vi "reference point (SubVI).vi"(0 "Nb Circles (Circle Detection 1)":i32, 1 "Straight Edge (Find Straight Edge 1)":T1, 2 "Straight Edge (Find Straight Edge 2)":T1, 3 "Particle Measurements (Real-World) (Particle Analysis 1)":dbl[][](array[numeric]) format="%.2f") -> (5 "Puck X, Y co-ordinates":dbl[][](array[numeric]), 6 "Player X, Y co-ordinates":dbl[][](array[numeric]))   [LabVIEW 2013]
uses:
  <vilib>/vision/NI_Vision_Development_Module.lvlib
panel:
  out "Reference Point in real\n (intersection)":cluster{"X":sgl, "Y":sgl} {"Y" format="%.2f"; "X" format="%.2f"}
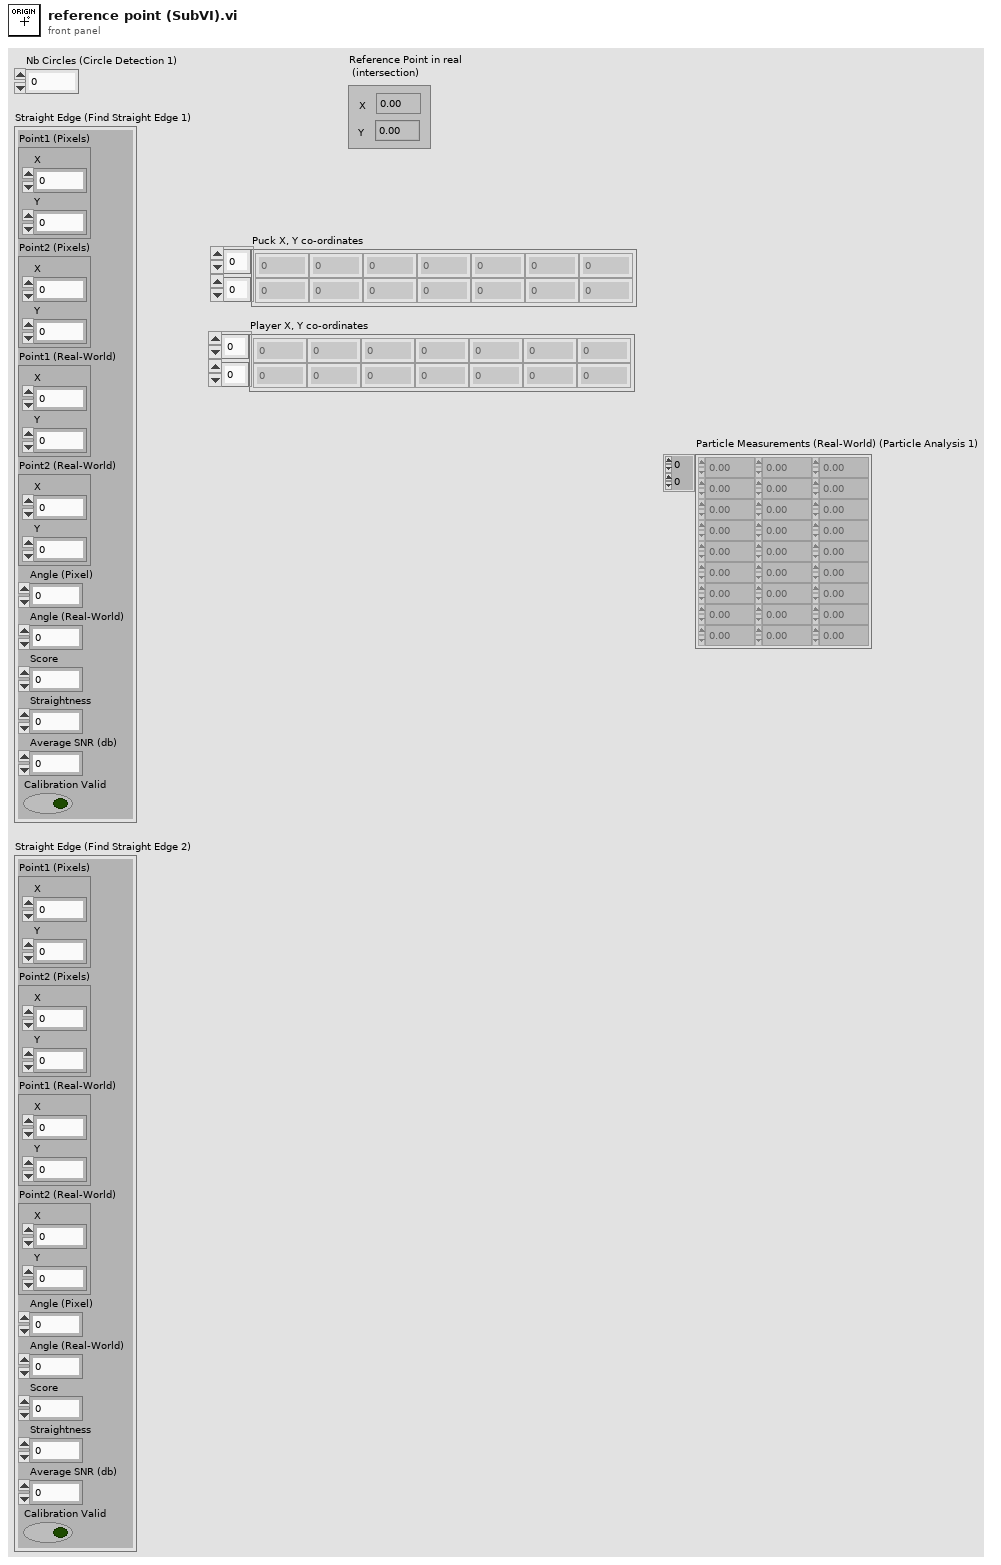
[diagram p1: front panel]
types:
  T1 = cluster{"Point1 (Pixels)":cluster{"X":sgl, "Y":sgl}, "Point2 (Pixels)":cluster{"X":sgl, "Y":sgl}, "Point1 (Real-World)":cluster{"X":sgl, "Y":sgl}, "Point2 (Real-World)":cluster{"X":sgl, "Y":sgl}, "Angle (Pixel)":dbl, "Angle (Real-World)":dbl, "Score":dbl, "Straightness":dbl, "Average SNR (db)":dbl, "Calibration Valid":bool}
  T2 = cluster{"Point1 (Real-World)":cluster{"X":sgl, "Y":sgl}, "Point2 (Real-World)":cluster{"X":sgl, "Y":sgl}}
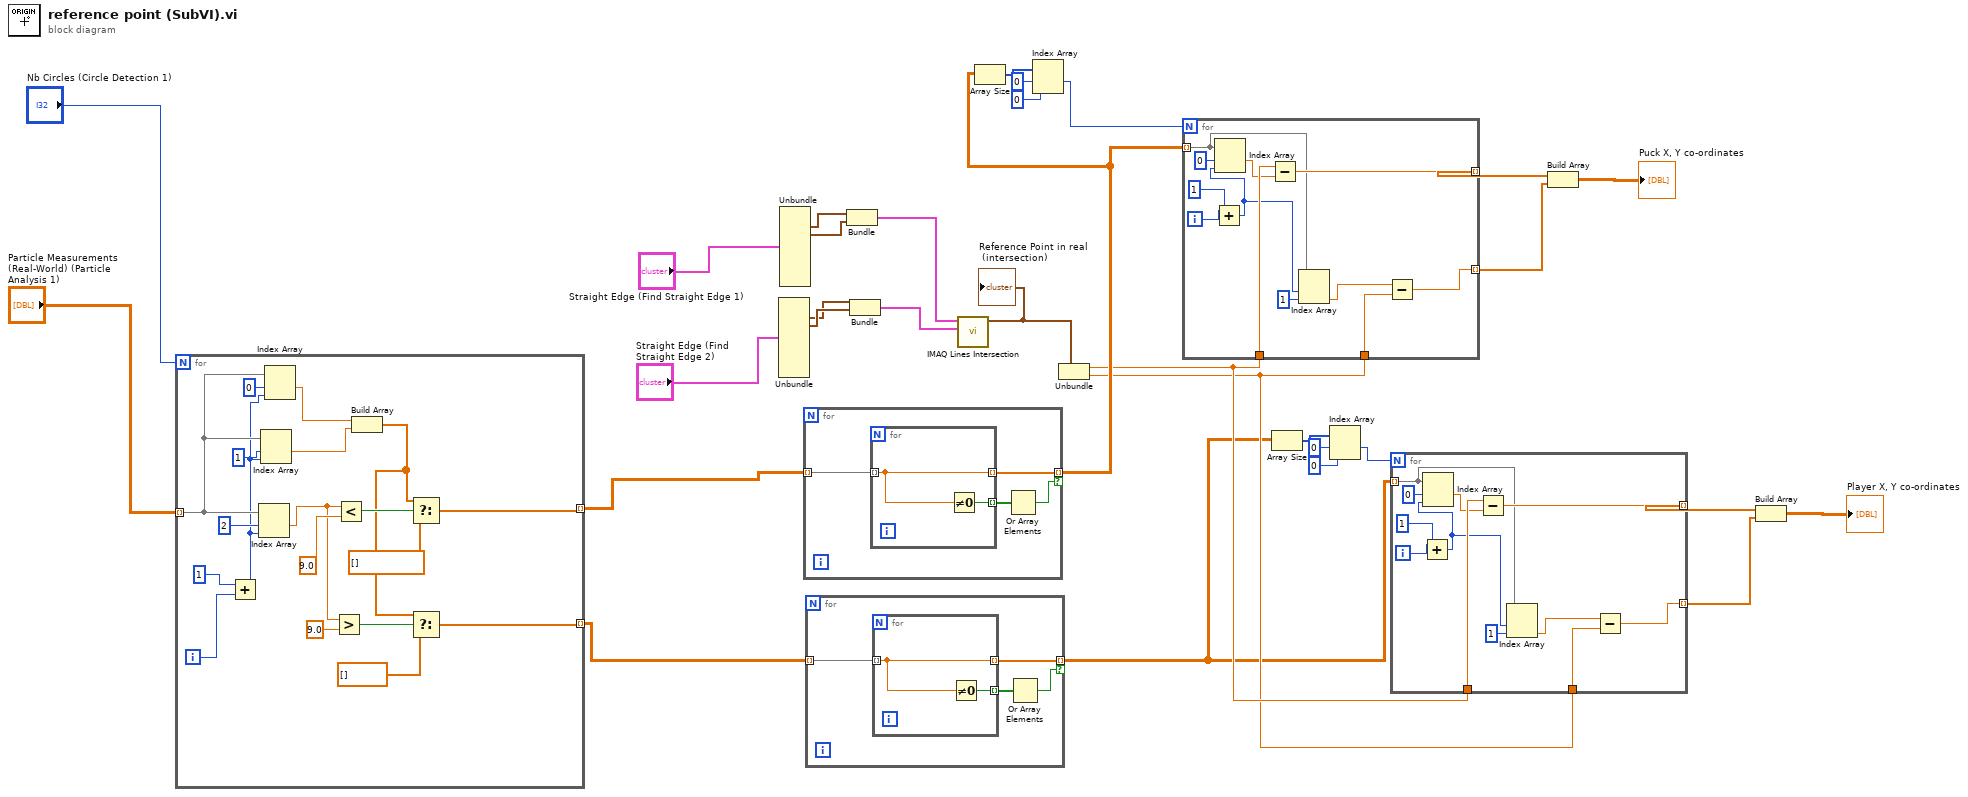
[diagram p0: block diagram]
diagram:
  n1 = for {
    N: "Nb Circles (Circle Detection 1)" -> [_]
    tunnel: "Particle Measurements (Real-World) (Particle Analysis 1)" -> [w43] mode=indexing
    tunnel: [w45] -> w18 mode=indexing
    tunnel: [w32] -> w17 mode=indexing
    i -> [w49]
    n2 = Add(x=1, y=w49) -> (x+y=w41:i32)
    n3 = Index Array(array=w43, index #1=2 ("index"), index #2=w41) -> (element #1=w36:dbl)  [unwired: 1 out]
    n4 = Index Array(array=w43, index #1=1 ("index"), index #2=w41) -> (element #1=w39:dbl)  [unwired: 1 out]
    n5 = Index Array(array=w43, index #1=0 ("index"), index #2=w41) -> (element #1=w40:dbl)  [unwired: 1 out]
    n6 = Greater?(x=w36, y=9.0) -> (0:w35:bool)
    n7 = Less?(x=w36, y=9.0) -> (x < y?=w46:bool)
    n8 = Build Array(w40, w39) -> (w34:dbl[])
    n9 = Select(t=w34, s=w46, f=dbl[] []) -> (s? t:f=w45:dbl[])
    n10 = Select(t=w34, s=w35, f=dbl[] []) -> (s? t:f=w32:dbl[])
  }
  n11 = Unbundle("Straight Edge (Find Straight Edge 2)") -> ("Point1 (Real-World)"=w23:cluster{"X":sgl, "Y":sgl}, "Point2 (Real-World)"=w24:cluster{"X":sgl, "Y":sgl})  [unwired: 8 out]
  n12 = Unbundle("Straight Edge (Find Straight Edge 1)") -> ("Point1 (Real-World)"=w26:cluster{"X":sgl, "Y":sgl}, "Point2 (Real-World)"=w25:cluster{"X":sgl, "Y":sgl})  [unwired: 8 out]
  n13 = for {
    tunnel: w18 -> [w54] mode=indexing
    tunnel: [w52] -> w15 mode=indexing if=w51
    n14 = for {
      tunnel: w54 -> [w55] mode=indexing
      tunnel: [w56] -> w53 mode=indexing
      tunnel: [w55] -> w52 mode=indexing
      n15 = Not Equal To 0?(x=w55) -> (x != 0?=w56:bool)
    }
    n16 = Or Array Elements(Boolean array=w53) -> (logical OR=w51:bool)
  }
  n17 = for {
    tunnel: w17 -> [w60] mode=indexing
    tunnel: [w58] -> w1 mode=indexing if=w57
    n18 = for {
      tunnel: w60 -> [w61] mode=indexing
      tunnel: [w62] -> w59 mode=indexing
      tunnel: [w61] -> w58 mode=indexing
      n19 = Not Equal To 0?(x=w61) -> (x != 0?=w62:bool)
    }
    n20 = Or Array Elements(Boolean array=w59) -> (logical OR=w57:bool)
  }
  n21 = Bundle("Point1 (Real-World)"=w26, "Point2 (Real-World)"=w25) -> (w30:T2)  [unwired: 1 in]
  n22 = Bundle("Point1 (Real-World)"=w23, "Point2 (Real-World)"=w24) -> (w28:T2)  [unwired: 1 in]
  n23 = call "IMAQ Lines Intersection"("Line 2"=w28, "Line 1"=w30) -> ("Intersection Point"=w31:cluster{"X":sgl, "Y":sgl})  [unwired: 7 in, 2 out]
  "Reference Point in real\n (intersection)" <- w31
  n24 = Array Size(array=w15) -> (size(s)=w14:i32[])
  n25 = Index Array(array=w14, index #1=0 ("index"), index #2=0 ("index")) -> (element #1=w11:i32)  [unwired: 1 out]
  n26 = Unbundle(w31) -> ("X"=w7:sgl, "Y"=w6:sgl)
  n27 = for {
    N: w11 -> [_]
    tunnel: w15 -> [w68] mode=indexing
    tunnel: w7 -> [w74]
    tunnel: [w72] -> w22 mode=indexing
    tunnel: [w63] -> w21 mode=indexing
    tunnel: w6 -> [w65]
    i -> [w70]
    n28 = Add(x=w70, y=1) -> (x+y=w66:i32)
    n29 = Index Array(array=w68, index #1=0 ("index"), index #2=w66) -> (element #1=w73:dbl)  [unwired: 1 out]
    n30 = Subtract(x=w74, y=w73) -> (x-y=w72:dbl)
    n31 = Index Array(array=w68, index #1=w66, index #2=1 ("index")) -> (element #2=w64:dbl)  [unwired: 1 out]
    n32 = Subtract(x=w64, y=w65) -> (x-y=w63:dbl)
  }
  n33 = Array Size(array=w1) -> (size(s)=w3:i32[])
  n34 = Index Array(array=w3, index #1=0 ("index"), index #2=0 ("index")) -> (element #1=w2:i32)  [unwired: 1 out]
  n35 = for {
    N: w2 -> [_]
    tunnel: w1 -> [w80] mode=indexing
    tunnel: w7 -> [w86]
    tunnel: [w84] -> w8 mode=indexing
    tunnel: [w75] -> w9 mode=indexing
    tunnel: w6 -> [w77]
    i -> [w82]
    n36 = Add(x=w82, y=1) -> (x+y=w78:i32)
    n37 = Index Array(array=w80, index #1=0 ("index"), index #2=w78) -> (element #1=w85:dbl)  [unwired: 1 out]
    n38 = Subtract(x=w86, y=w85) -> (x-y=w84:dbl)
    n39 = Index Array(array=w80, index #1=w78, index #2=1 ("index")) -> (element #2=w76:dbl)  [unwired: 1 out]
    n40 = Subtract(x=w76, y=w77) -> (x-y=w75:dbl)
  }
  n41 = Build Array(w22, w21) -> (→"Puck X, Y co-ordinates":dbl[][])
  n42 = Build Array(w8, w9) -> (→"Player X, Y co-ordinates":dbl[][])
